vi "Grid Measurements with VISA connection to user instrument.vi"(6 "Internal use":string, 7 "Grid param":T1 {"height (m)" format="%#_6p"; "width (m)" format="%#_6p"; "center Y (m)" format="%#_6p"; "center X (m)" format="%#_6p"}, 8 "Error in (no error)":errorcluster, 9 "Points Y/Index Y":i32, 10 "Points X/Index X":i32, 11 "Method":enum16{"init", "run", "end"}(ring)) -> (0 "Error out":errorcluster)   [LabVIEW 2017]
doc: "Example of a measurement VI to be used in the \"Experiments on a Grid\" tool as external VI.\n\n- Nanonis Programming Interface -"
uses:
  Nanonis Prog Interface.lvlib
panel:
  # "Example VI for use with the \"Experiments on a Grid\" module.\n\n\"Experiments on a Grid\" will first (before starting the measurements) call the external VI with the \"init\" method, passing the grid resolution (Points X, Points Y) and the grid dimensions (Grid).\nThen, for the measurements, the external VI will be called with the \"run\" method, passing the current X and Y indices (Index X, Index Y).\nAfter the last measurement, the external VI will be called using the \"end\" method."
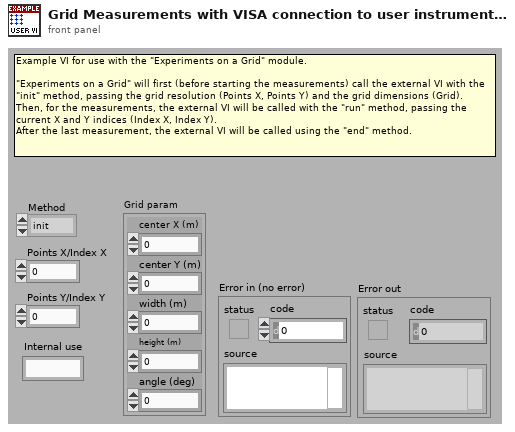
[diagram p1: front panel]
types:
  T1 = cluster{"center X (m)":sgl, "center Y (m)":sgl, "width (m)":sgl, "height (m)":sgl, "angle (deg)":sgl}
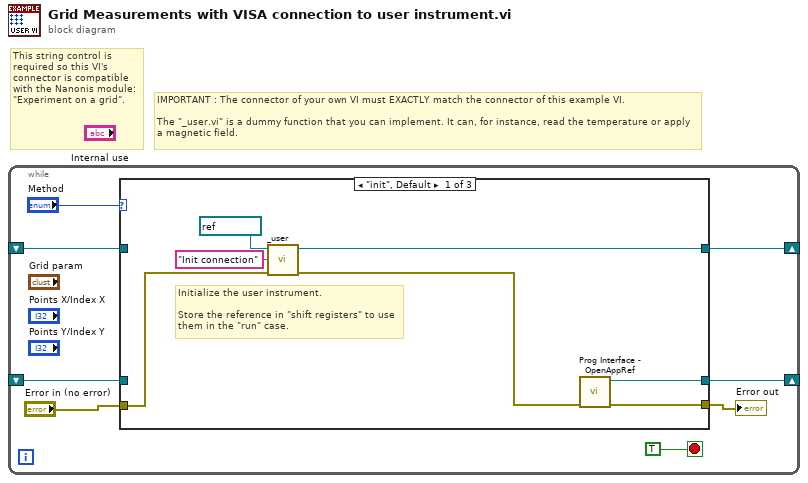
[diagram p0: block diagram]
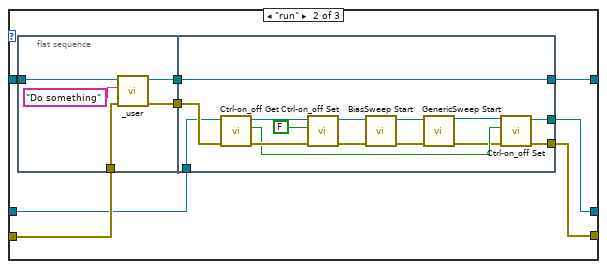
[diagram p2: hidden frame]
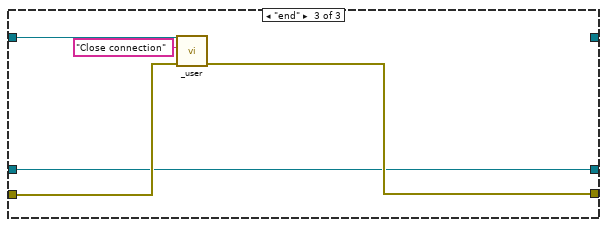
[diagram p3: hidden frame]
diagram:
  # "This string control is required so this VI's connector is compatible with the Nanonis module: \"Experiment on a grid\"."
  # "IMPORTANT : The connector of your own VI must EXACTLY match the connector of this example VI.\n\nThe \"_user.vi\" is a dummy function that you can implement. It can, for instance, read the temperature or apply\na magnetic field."
  n1 = while {
    shift-right: [w6] -> _
    shift-left: _ -> [w5]
    shift-right: [w2] -> _
    shift-left: _ -> [w1]
    stop <- TRUE stop-if-true
    n2 = case shown="\"init\", Default" "Method" {
      tunnel: [w14 w22 _] -> w6
      tunnel: w5 -> [_ w23 w48]
      tunnel: "Error in (no error)" -> [w15 w20 w46]
      tunnel: [w10 w21 w45] -> w3
      tunnel: [w9 w16 w44] -> w2
      tunnel: w1 -> [_ w17 w44]
      frame "init", Default {
        # "Initialize the user instrument. \n\nStore the reference in \"shift registers\" to use them in the \"run\" case."
        n3 = call "_user.vi"("error in (no error)"=w15, "Send"="Init connection", "VISA resource name"=refnum<visa-resource-name> "COM1") -> ("error out"=w11:errorcluster, "VISA resource name"=w14:refnum<visa-resource-name>)  [unwired: 6 in, 1 out]
        n4 = call <userlib>:"Prog Interface - OpenAppRef.vi"("Error in (no error)"=w11) -> ("Error out"=w10:errorcluster, "Application reference"=w9:refnum<vi>)  [unwired: 5 in]
      }
      frame "run" {
        n5 = flat-sequence {
          tunnel: w23 -> [w28]
          tunnel: w20 -> [w25]
          tunnel: [w27] -> w19
          tunnel: [w26] -> w18
          tunnel: [w43] -> w22
          tunnel: w19 -> [w43]
          tunnel: [w36] -> w21
          tunnel: w18 -> [w35]
          tunnel: w17 -> [w34]
          tunnel: [w29] -> w16
          frame #0 {
            n6 = call "_user.vi"("error in (no error)"=w25, "Send"="Do something" ("write buffer"), "VISA resource name"=w28) -> ("error out"=w26:errorcluster, "VISA resource name"=w27:refnum<visa-resource-name>)  [unwired: 6 in, 1 out]
          }
          frame #1 {
            n7 = call <userlib>:"Ctrl-on_off Get.vi"("error in (no error)"=w35, "Application ref in"=w34) -> ("error out"=w41:errorcluster, "Z-Controller on/off status"=w40:bool, "Application ref out"=w33:refnum<vi>)  [unwired: 7 in]
            n8 = call <userlib>:"Ctrl-on_off Set.vi"("error in (no error)"=w41, "Z Controller ON/OFF"=FALSE ("Ctrl on/off"), "Application ref in"=w33) -> ("error out"=w39:errorcluster, "Application ref out"=w32:refnum<vi>)  [unwired: 7 in]
            n9 = call <userlib>:"BiasSweep Start.vi"("Error in (no error)"=w39, "Application ref in"=w32) -> ("Error out"=w38:errorcluster, "Application ref out"=w31:refnum<vi>)  [unwired: 6 in, 2 out]
            n10 = call <userlib>:"GenericSweep Start.vi"("Application ref in"=w31, "error in (no error)"=w38) -> ("Application ref out"=w30:refnum<vi>, "error out"=w37:errorcluster)  [unwired: 10 in, 2 out]
            n11 = call <userlib>:"Ctrl-on_off Set.vi"("error in (no error)"=w37, "Z Controller ON/OFF"=w40, "Application ref in"=w30) -> ("error out"=w36:errorcluster, "Application ref out"=w29:refnum<vi>)  [unwired: 7 in]
          }
        }
      }
      frame "end" {
        n12 = call "_user.vi"("error in (no error)"=w46, "Send"="Close connection", "VISA resource name"=w48) -> ("error out"=w45:errorcluster)  [unwired: 6 in, 2 out]
      }
    }
    "Error out" <- w3
  }
